vi "Dispose.vi"(8 "error in (no error)":errorcluster caption="错误输入（无错误）", 11 "同事（抽象） 输入":refnum<class "Colleague.lvclass"> caption="DNL_LabVIEW Object in") -> (0 "error out":errorcluster caption="错误输出", 3 "同事（抽象） 输出":refnum<class "Colleague.lvclass"> caption="DNL_LabVIEW Object out")   [LabVIEW 2011, in "Colleague.lvclass"]
uses:
  Colleague.lvclass
  Colleague.lvclass/Colleague.ctl
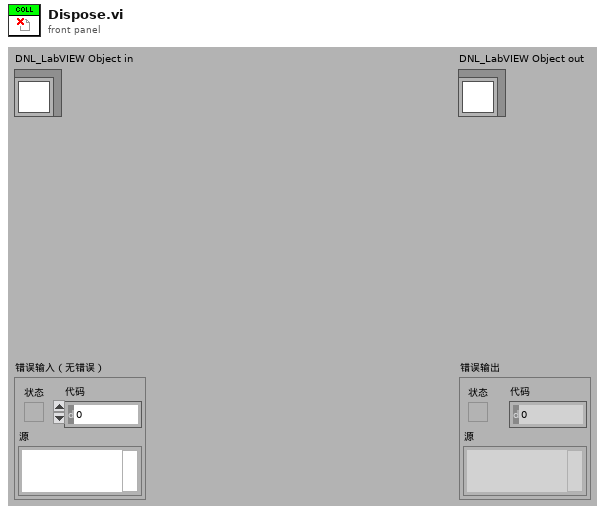
[diagram p1: front panel]
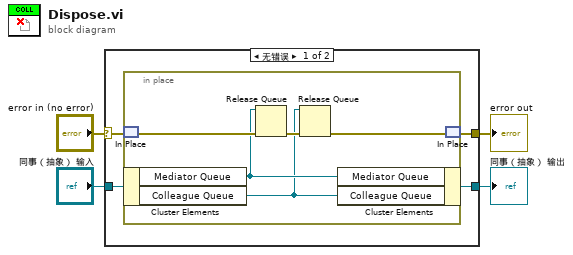
[diagram p0: block diagram]
diagram:
  n1 = case shown="无错误" "error in (no error)" {
    selector: "error in (no error)" -> [w6 w15]
    tunnel: [w5 w15] -> w3
    tunnel: [w7 w14] -> w1
    tunnel: "同事（抽象） 输入" -> [w8 w14]
    frame No Error {
      n2 = in-place {
        n3 = in-place-match #1(w6) -> (w13:errorcluster)
        n4 = in-place-cluster #2(w8) -> ("Mediator Queue"=w10:refnum<queue>, "Colleague Queue"=w9:refnum<queue>)
        n5 = Release Queue(queue=w10, error in (no error)=w13) -> (error out=w12:errorcluster)  [unwired: 1 in, 2 out]
        n6 = Release Queue(queue=w9, error in (no error)=w12) -> (error out=w11:errorcluster)  [unwired: 1 in, 2 out]
        n7 = in-place-cluster #2("Mediator Queue"=w10, "Colleague Queue"=w9) -> (w7:refnum<class "Colleague.lvclass">)
        n8 = in-place-match #1(w11) -> (w5:errorcluster)
      }
    }
    frame Error {
    }
  }
  "error out" <- w3
  "同事（抽象） 输出" <- w1
